vi "DHE_DescribeDriverErrors.vi"(0 "message":string, 2 "OK message":string="DONE", 3 "error in (no error)":errorcluster) -> (7 "error?":bool, 8 "astroerrors":string, 10 "error out":errorcluster)   [LabVIEW 2016]
doc: "This subVI tests the error status output of one or more low-level functions or subVIs that output a numeric error code, and creates an error out cluster that can be wired to the Simple or General Error Handler in order to identify the error and describe it to the user.\n\nThe error in cluster is tested first. If error? is no-error, the elements of the error codes array are tested next for non-zero values. The first error found terminates the test, and error out identifies that error. Use a Build Array function to assemble the individual error codes.\n\nYou can optionally use the source messages string to pass on the source of the error. Enter one line of text for each element of the error codes array. \n\nThe error? status is TRUE on any error."
uses:
  expglobal.vi
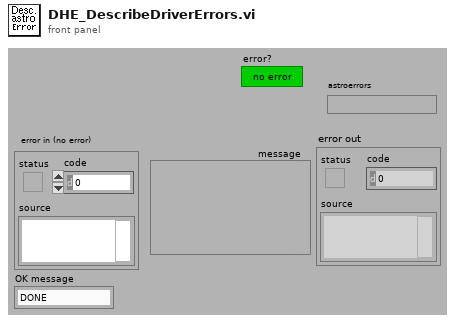
[diagram p1: front panel]
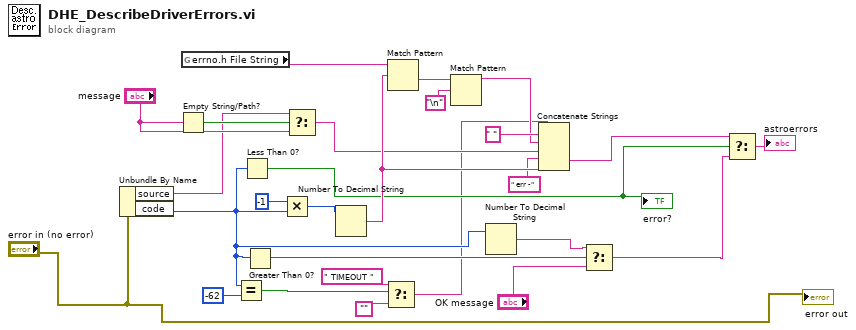
[diagram p0: block diagram]
diagram:
  n1 = Unbundle By Name("error in (no error)") -> ("source"=w15:string, "code"=w11:i32)
  n2 = Empty String/Path?(string/path="message") -> (empty?=w17:bool)
  n3 = global read "expglobal.vi" "errno.h File String"() -> (w21:string)
  n4 = Equal?(x=w11, y=-62) -> (x = y?=w9:bool)
  n5 = Less Than 0?(x=w11) -> (x < 0?=w19:bool)
  "error?" <- w19
  n6 = Greater Than 0?(x=w11) -> (x > 0?=w12:bool)
  n7 = Multiply(x=-1, y=w11) -> (x*y=w1:i32)
  n8 = Select(t=w15, s=w17, f="message") -> (s? t:f=w14:string)
  n9 = Number To Decimal String(number=w1) -> (decimal integer string=w23:string)  [unwired: 1 in]
  n10 = Select(t=" TIMEOUT ", s=w9, f="") -> (s? t:f=w6:string)
  n11 = Match Pattern(string=w21, regular expression=w23) -> (after substring=w25:string)  [unwired: 1 in, 3 out]
  n12 = Match Pattern(string=w25, regular expression="\n") -> (before substring=w13:string)  [unwired: 1 in, 3 out]
  n13 = Number To Decimal String(number=w11) -> (decimal integer string=w2:string)  [unwired: 1 in]
  n14 = Concatenate Strings(w6, " ", w13, w14, " err -", w23) -> (w27:string)
  n15 = Select(t=w2, s=w12, f="OK message") -> (s? t:f=w4:string)
  n16 = Select(t=w27, s=w19, f=w4) -> (s? t:f=→"astroerrors":string)
  "error out" <- "error in (no error)"
